vi "GV trigger output preset.vi"() -> ()   [LabVIEW 2017]
panel:
  out "TriggerOutputPreset":bool
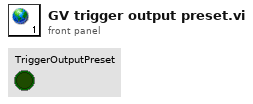
[diagram p1: front panel]
diagram:
